vi "Create Single Element Packed Info.vi"(11 "Single Element":T5) -> (3 "Packed Data Encoding":T1)   [LabVIEW 2021, in "CIF_NI_CIPC.lvlib"]
doc: "When individual elements are read individually from a larger structure, this will create the packed data encoding for that element."
uses:
  CIF_NI_CIPC.lvlib
  TypeDefs/Data Element.ctl
  <vilib>/Utility/Data Type/Type Definitions/Data Type.ctl
  TypeDefs/Data Encoding.ctl
  TypeDefs/Alignment.ctl
  <vilib>/CIF Foundation/CIF Utilities/DataTypes/Typedef/Endian.ctl
  TypeDefs/Data Struct Array Info.ctl
  <vilib>/CIF Foundation/CIF Utilities/DataTypes/DataTypes_CIF_U.lvlib
  <vilib>/Utility/Data Type/NI_Data Type.lvlib
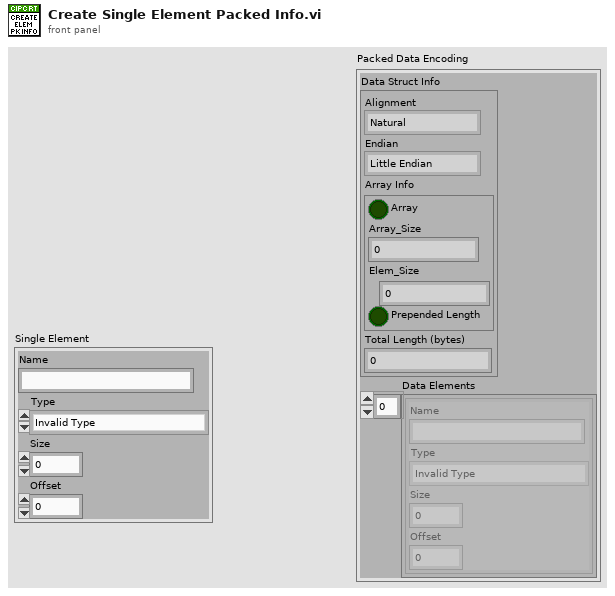
[diagram p1: front panel]
types:
  T1 = typedef "CIF_NI_CIPC.lvlib/Data Encoding.ctl" = cluster{"Data Struct Info":cluster{"Alignment":T2, "Endian":T3, "Array Info":T4, "Total Length (bytes)":i32}, "Data Elements":T5[]}
  T2 = typedef "CIF_NI_CIPC.lvlib/Alignment.ctl" = enum16{"Natural", "Packed"}
  T3 = typedef "DataTypes_CIF_U.lvlib/Endian.ctl" = enum16{"Little Endian", "Big Endian"}
  T4 = typedef "CIF_NI_CIPC.lvlib/Data Struct Array Info.ctl" = cluster{"Array":bool, "Array_Size":i32, "Elem_Size":i32, "Prepended Length":bool}
  T5 = typedef "CIF_NI_CIPC.lvlib/Data Element.ctl" = cluster{"Name":string, "Type":T6, "Size":u32, "Offset":u32}
  T6 = typedef "NI_Data Type.lvlib/Data Type.ctl" = enum8{"Invalid Type", "Void", "I8", "I16", "I32", "I64", "U8", "U16", "U32", "U64", "Single Float", "Double Float", "Extended Float", "Single Complex", "Double Complex", "Extended Complex", "Enum U8", "Enum U16", "Enum U32", "Enum U64", "Single Float With Unit", "Double Float With Unit", "Extended Float With Unit", "Single Complex with Unit", "Double Complex with Unit", "Extended Complex with Unit", "Boolean", "String", "Path", "Picture", "Tag", "Array", "Cluster", "Variant", "LV Variant", "Waveform", "Timestamp", "Digital Waveform", "Digital Data", "ExpressData", "Refnum", "External Data", "VI", "Poly VI", "LabVIEW Class Instance", "Fixed Point", "Set Collection", "Map Collection"}
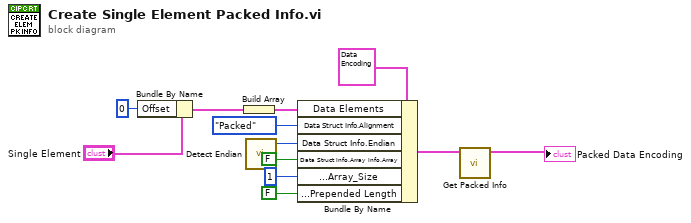
[diagram p0: block diagram]
diagram:
  n1 = Bundle By Name(cluster="Single Element", "Offset"=u32 0) -> (w6:T5)
  n2 = Build Array(w6) -> (w11:T5[])
  n3 = call <vilib>:"Detect Endian.vi"() -> ("Endian"=w4:T3)  [unwired: 5 in]
  n4 = Bundle By Name(cluster=T1 {"Data Struct Info"={"Alignment"=enum."Packed", "Endian"=enum."Little Endian", "Array Info"={"Array"=FALSE, "Array_Size"=0, "Elem_Size"=0, "Prepended Length"=FALSE}, "Total Length (bytes)"=0}, "Data Elements"=[]} ("Packed Data Encoding"), "Data Elements"=w11, "Data Struct Info.Alignment"=Alignment."Packed", "Data Struct Info.Endian"=w4, "Data Struct Info.Array Info.Array"=FALSE, "Data Struct Info.Array Info.Array_Size"=1, "Data Struct Info.Array Info.Prepended Length"=FALSE) -> (w10:T1)
  n5 = call "Get Packed Info.vi"("Data Encoding In"=w10) -> ("Packed Data Encoding"=→"Packed Data Encoding":T1)  [unwired: 10 in]
